vi "multimetr.vi"() -> (3 "read buffer":string)   [LabVIEW 2018]
doc: "Wymusza pomiar mulitmetrem"
uses:
  Open_device_2017.llb/Select_Instr.ctl
panel:
  out "error out":errorcluster
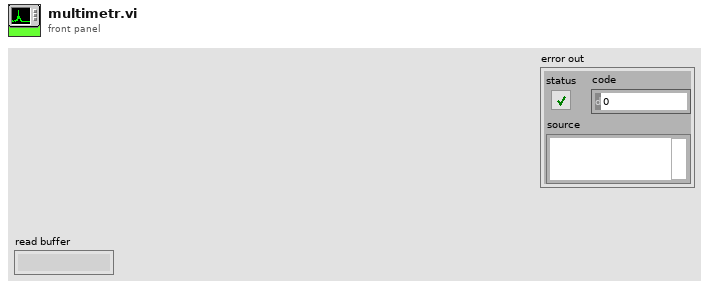
[diagram p1: front panel]
types:
  T1 = typedef "Select_Instr.ctl" = string
  T2 = cluster{"VISA resource name":refnum<visa-resource-name>}
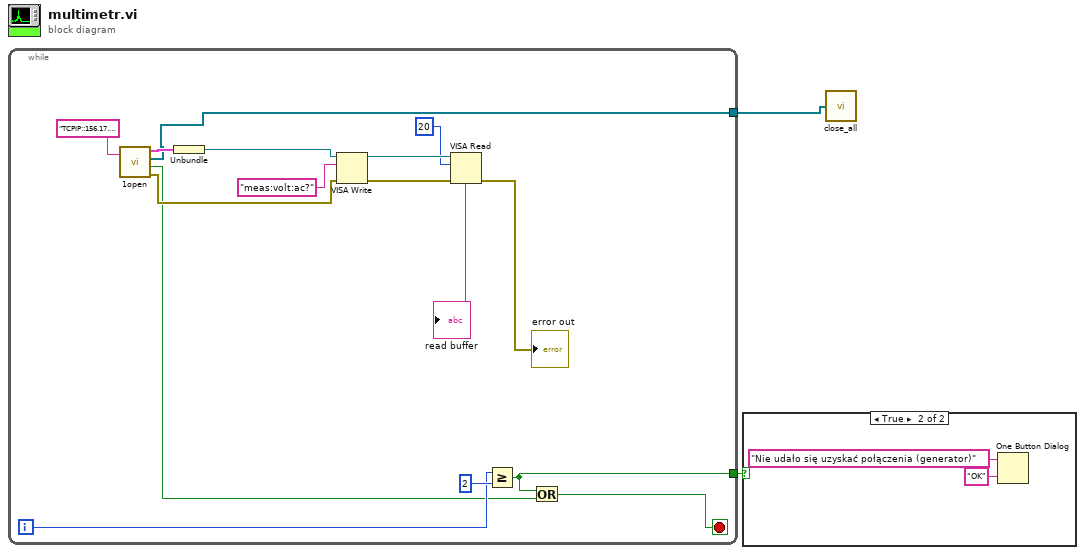
[diagram p0: block diagram]
diagram:
  n1 = while {
    tunnel: [w8] -> w2
    tunnel: [w3] -> w1
    i -> [w5]
    stop <- w6 stop-if-true
    n2 = call "1open.vi"("VISA resource name"=T1 "TCPIP::156.17.45.35::inst27::INSTR" ("Select_Instrument")) -> ("InstrCluster"=w17:T2, "InstrArray"=w8:refnum<visa-resource-name>[], "Open OK (true)"=w4:bool, "error out"=w9:errorcluster)  [unwired: 1 in]
    n3 = Unbundle(w17) -> ("VISA resource name"=w16:refnum<visa-resource-name>)
    n4 = VISA Write(VISA resource name=w16, write buffer="meas:volt:ac?", error in (no error)=w9) -> (VISA resource name out=w14:refnum<visa-resource-name>, error out=w12:errorcluster)  [unwired: 1 out]
    n5 = VISA Read(VISA resource name=w14, byte count=20, error in (no error)=w12) -> (read buffer=→"read buffer":string, error out=→"error out":errorcluster)  [unwired: 2 out]
    n6 = Greater Or Equal?(x=w5, y=2) -> (x >= y?=w3:bool)
    n7 = Or(x=w3, y=w4) -> (x .or. y?=w6:bool)
  }
  n8 = case shown="True" w1 {
    frame False {
    }
    frame True {
      n9 = One Button Dialog(message="Nie udało się uzyskać połączenia (generator)", button name ("OK")="OK") -> ()  [unwired: 1 out]
    }
  }
  n10 = call "close_all.vi"("OpenRes"=w2) -> ()  [unwired: 1 out]
